vi "CalculateAmply.vi"(10 "image":sgl, 11 "real":sgl) -> (3 "amply":dbl)   [LabVIEW 2012]
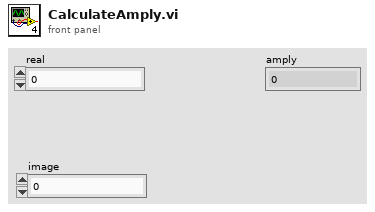
[diagram p1: front panel]
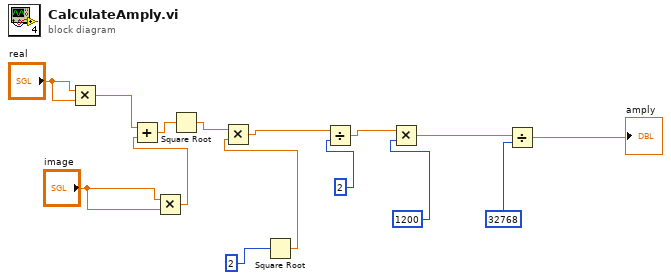
[diagram p0: block diagram]
diagram:
  n1 = Multiply(x="real", y="real") -> (x*y=w13:sgl)
  n2 = Multiply(x="image", y="image") -> (x*y=w12:sgl)
  n3 = Add(x=w13, y=w12) -> (x+y=w11:sgl)
  n4 = Square Root(x=w11) -> (sqrt(x)=w10:sgl)
  n5 = Square Root(x=2) -> (sqrt(x)=w8:dbl)
  n6 = Multiply(x=w10, y=w8) -> (x*y=w6:dbl)
  n7 = Divide(x=w6, y=2) -> (x/y=w5:dbl)
  n8 = Multiply(x=w5, y=1200) -> (x*y=w3:dbl)
  n9 = Divide(x=w3, y=32768) -> (x/y=→"amply":dbl)
